vi "xijk_select_best_filter.vi"(7 "spectra parameters in":T1={"Booleans"={"Notch filtering"=FALSE, "Unknown detector"=FALSE, "Dual band filters"=FALSE, "Dual emission by cubes"=FALSE, "FRET"=FALSE}, "Integers"={"Light source"=0, "Number of fluorophores"=0, "Wavelength of laser (nm) 1"=0, "Broadness of laser (nm) 1"=0.0, "Wavelength of laser (nm) 2"=0, "Broadness of laser (nm) 2"=0.0, "Template"=1}, "Doubles"={"Molar extinction 1"=1.0, "Molar extinction 2"=1.0, "Quantum efficiency 1"=1.0, "Quantum efficiency 2"=1.0}}, 8 "error in":errorcluster, 9 "calculation table":i32[](array[numeric])=[8, 15, 13, 10], 10 "Column Sort Order":i32[](array[numeric])=[8, 15], 11 "file to be analyzed":path) -> (0 "error out":errorcluster, 1 "sorted output paths table":string[][](array[string]))   [LabVIEW 2010, in "xijk_select_best_filter.lvlib"]
uses:
  xijk_select_best_filter.lvlib
  Type Def/spectra_parameters.ctl
  <vilib>/Utility/file.llb/Read From Spreadsheet File (string).vi
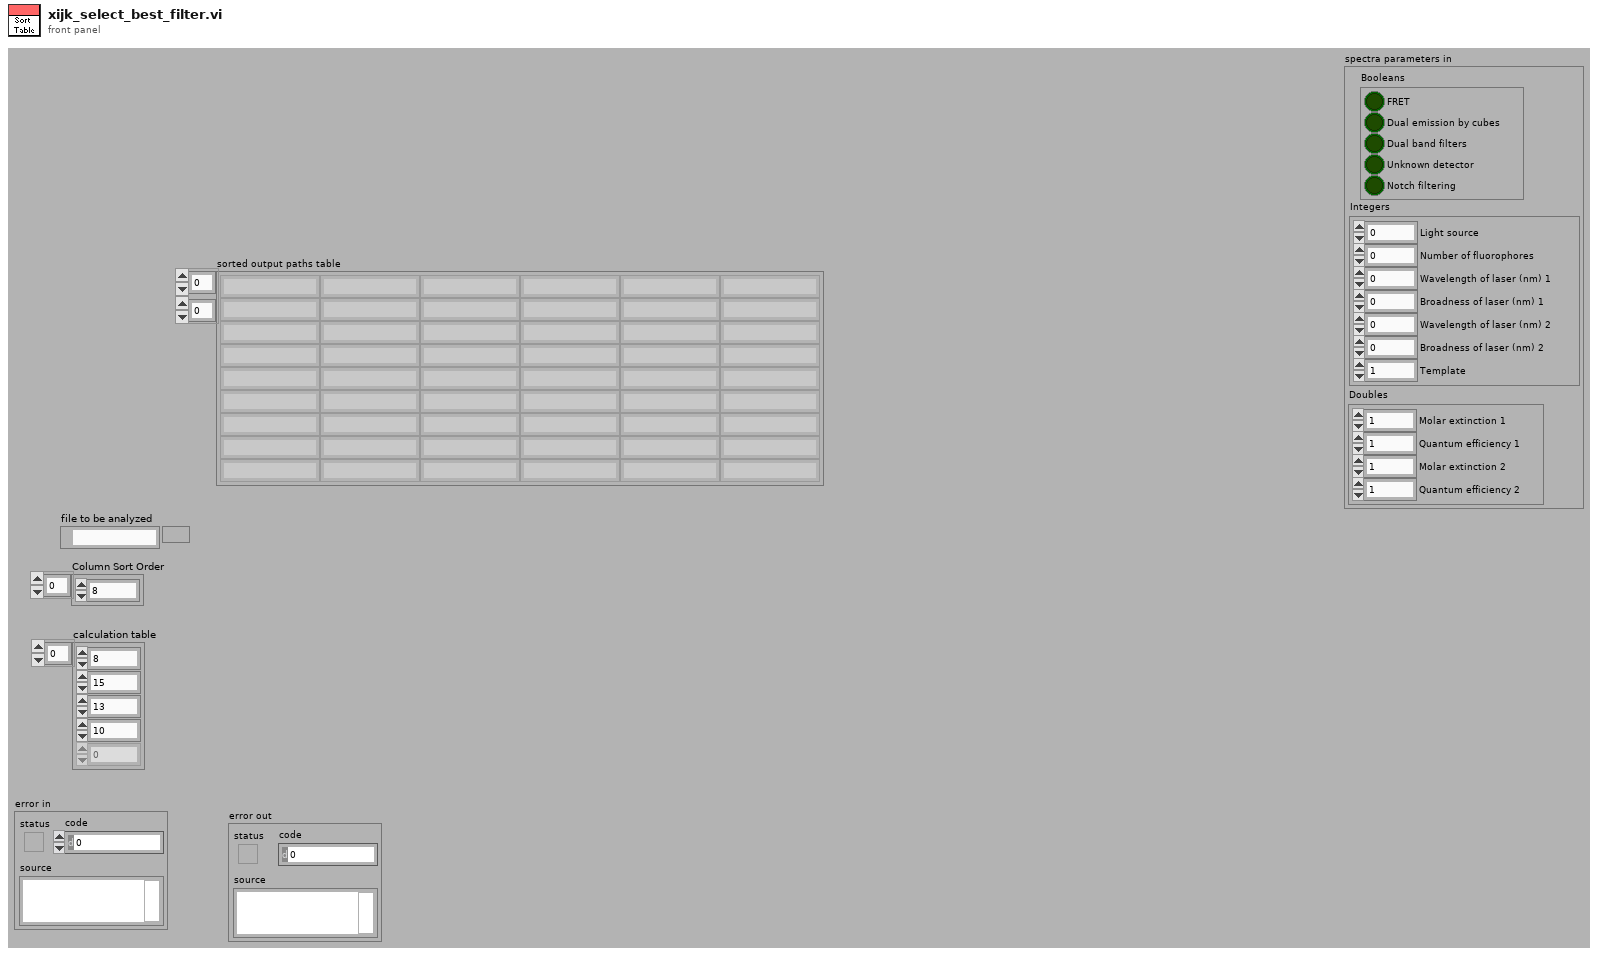
[diagram p1: front panel]
types:
  T1 = typedef "spectra_parameters.ctl" = cluster{"Booleans":cluster{"Notch filtering":bool, "Unknown detector":bool, "Dual band filters":bool, "Dual emission by cubes":bool, "FRET":bool}, "Integers":cluster{"Light source":u16, "Number of fluorophores":u16, "Wavelength of laser (nm) 1":u16, "Broadness of laser (nm) 1":sgl, "Wavelength of laser (nm) 2":u16, "Broadness of laser (nm) 2":sgl, "Template":u16}, "Doubles":cluster{"Molar extinction 1":sgl, "Molar extinction 2":sgl, "Quantum efficiency 1":sgl, "Quantum efficiency 2":sgl}}
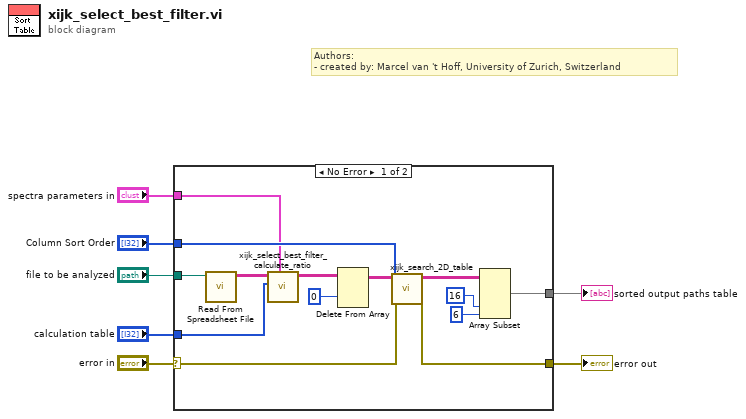
[diagram p0: block diagram]
diagram:
  # "Authors: \n- created by: Marcel van 't Hoff, University of Zurich, Switzerland"
  n1 = case shown="No Error" "error in" {
    selector: "error in" -> [w12 w22]
    tunnel: "file to be analyzed" -> [w21 _]
    tunnel: "Column Sort Order" -> [w20 _]
    tunnel: "calculation table" -> [w17 _]
    tunnel: [w11 w22] -> w3
    tunnel: [w15 _] -> w2
    tunnel: "spectra parameters in" -> [w8 _]
    frame No Error {
      n2 = call-poly <vilib>:"Read From Spreadsheet File.vi"("file path (dialog if empty)"=w21) -> ("all rows"=w19:string[][])  [unwired: 3 in, 7 out]
      n3 = call "xijk_select_best_filter_calculate_ratio.vi"("spectra parameters in"=w8, "calculation table"=w17, "all rows"=w19) -> ("all rows out"=w18:string[][])  [unwired: 8 out]
      n4 = Delete From Array(array=w18, index (row)=0) -> (array with subset deleted=w9:string[][])  [unwired: 2 in, 1 out]
      n5 = call "xijk_search_2D_table.vi"("error in"=w12, "sort array in"=w20, "all rows in"=w9) -> ("error out"=w11:errorcluster, "all rows out"=w13:string[][])  [unwired: 7 in]
      n6 = Array Subset(array=w13, index (col)=16 ("length"), length (col)=6 ("length")) -> (w15:string[][])  [unwired: 2 in]
    }
    frame Error {
    }
  }
  "error out" <- w3
  "sorted output paths table" <- w2
